vi "Exp_ICCD_GetAuxOutProperties.vi"(8 "error in (no error)":errorcluster, 11 "LightField Automation in":refnum<class "LightField Automation.lvclass">) -> (0 "error out":errorcluster, 1 "Aux Out Width (ns)":dbl, 2 "AuxOut Delay (ns)":dbl, 3 "LightField Automation out":refnum<class "LightField Automation.lvclass">)   [LabVIEW 2013, in "LightField Automation.lvclass"]
uses:
  LightField Automation.lvclass
  C:/Program Files/Princeton Instruments/LightField/PrincetonInstruments.LightFieldAddInSupportServices.dll
  Program Files/Princeton Instruments/LightField/PrincetonInstruments.LightFieldAddInSupportServices.dll
  LightField Automation.lvclass/LightField Automation.ctl
  C:/Program Files/Princeton Instruments/LightField/AddInViews/PrincetonInstruments.LightFieldViewV3.dll
  Program Files/Princeton Instruments/LightField/AddInViews/PrincetonInstruments.LightFieldViewV3.dll
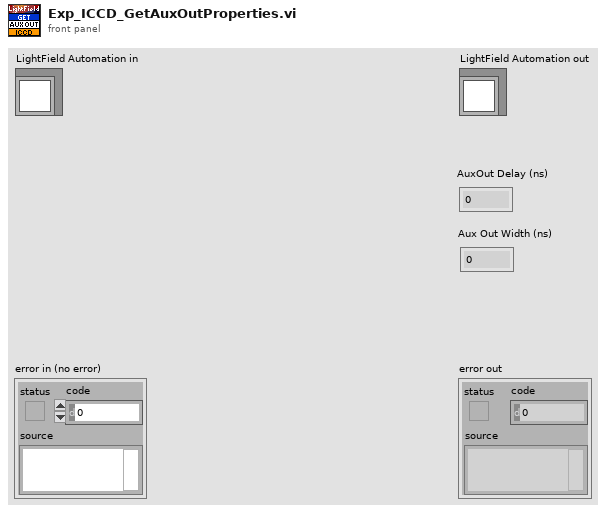
[diagram p1: front panel]
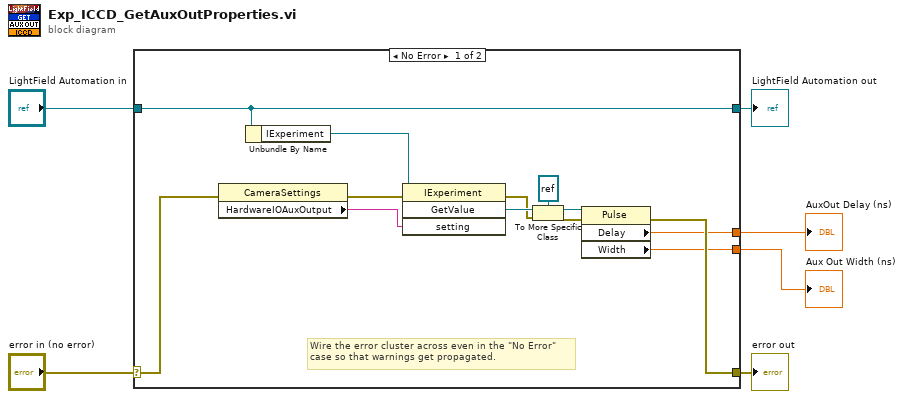
[diagram p0: block diagram]
diagram:
  n1 = case shown="No Error" "error in (no error)" {
    selector: "error in (no error)" -> [w17 w21]
    tunnel: [w9 w21] -> w5
    tunnel: [w19 w20] -> w3
    tunnel: "LightField Automation in" -> [w19 w20]
    tunnel: [w8 _] -> w2
    tunnel: [w7 _] -> w1
    frame No Error {
      # "Wire the error cluster across even in the \"No Error\"\ncase so that warnings get propagated."
      n2 = property class="CameraSettings"(error in=w17) -> (error out=w16:errorcluster, "HardwareIOAuxOutput"=w15:string)  [unwired: 1 in, 1 out]
      n3 = Unbundle By Name(w19) -> ("IExperiment"=w18:refnum<k24>)
      n4 = invoke class="IExperiment" method="GetValue"(reference=w18, error in=w16, "setting"=w15) -> (error out=w10:errorcluster, "GetValue"=w14:refnum<k24>)  [unwired: 1 in, 2 out]
      n5 = To More Specific Class(target class=refnum<k24> refnum ("reference out"), reference=w14, error in=w10) -> (specific class reference=w12:refnum<k24>, error out=w11:errorcluster)
      n6 = property class="Pulse"(reference=w12, error in=w11) -> (error out=w9:errorcluster, "Delay"=w8:dbl, "Width"=w7:dbl)  [unwired: 1 out]
    }
    frame Error {
    }
  }
  "error out" <- w5
  "LightField Automation out" <- w3
  "AuxOut Delay (ns)" <- w2
  "Aux Out Width (ns)" <- w1
